vi "FibrePhotometry.vi"() -> ()   [LabVIEW 2016]
uses:
  <vilib>/DAQmx/read.llb/DAQmx Read (Analog 2D DBL NChan NSamp).vi
  <vilib>/DAQmx/write.llb/DAQmx Write (Analog 1D DBL NChan 1Samp).vi
  <vilib>/DAQmx/miscellaneous.llb/DAQmx Fill In Error Info.vi
  <vilib>/Utility/file.llb/Write Delimited Spreadsheet (DBL).vi
  <vilib>/DAQmx/create/channels.llb/DAQmx Create Channel (AO-Voltage-Basic).vi
panel:
  out "Start Time":u32
  in  "Recording":bool
  out "Recording Time":dbl
  out "Save Path":path
  out "Data":dbl[][](graph)
  out "Waveform":waveform(dbl)[](graph)
  in  "stop":bool
  out "Loop Time":u32
  in  "Comments":string
  in  "Dir":string="C:\\Test"
  in  "Raw samples per s":dbl=2000.0 min=2000.0 max=2000.0
  in  "405 LED Power":dbl=1.0 min=0.0 max=5.0
  in  "470 LED power":dbl=2.0 min=0.0 max=5.0
  in  "Frequency":dbl=10.0
  in  "Duty cycle (%)":dbl=40.0
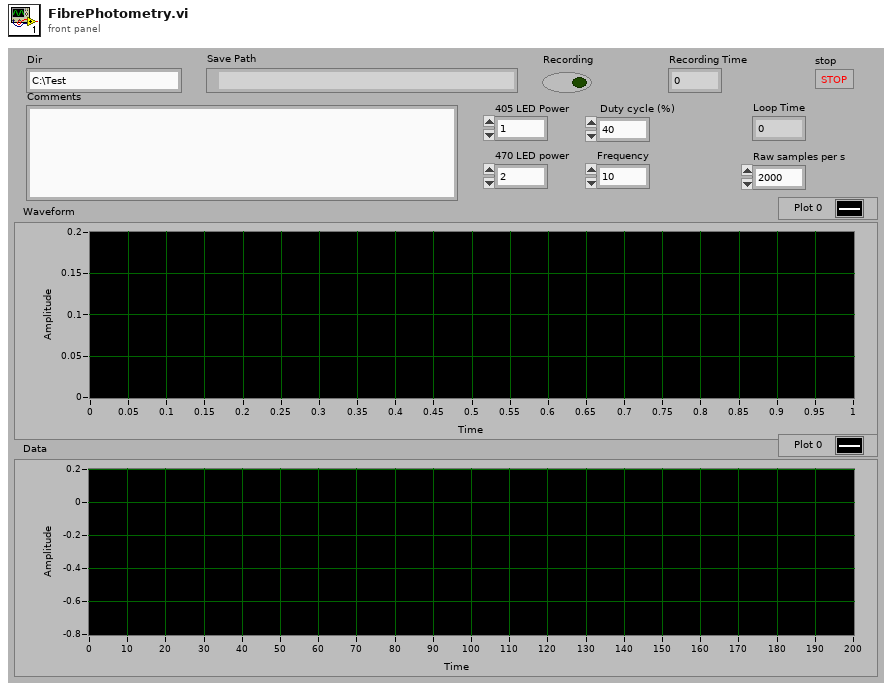
[diagram p1: front panel]
types:
  T1 = enum16{"big-endian, network order", "native, host order", "little-endian"}
  T2 = cluster{"Comments":string, "Dir":string, "Frequency":dbl, "470 LED power":dbl, "405 LED Power":dbl, "Raw samples per s":dbl, " Duty cycle (%)":dbl}
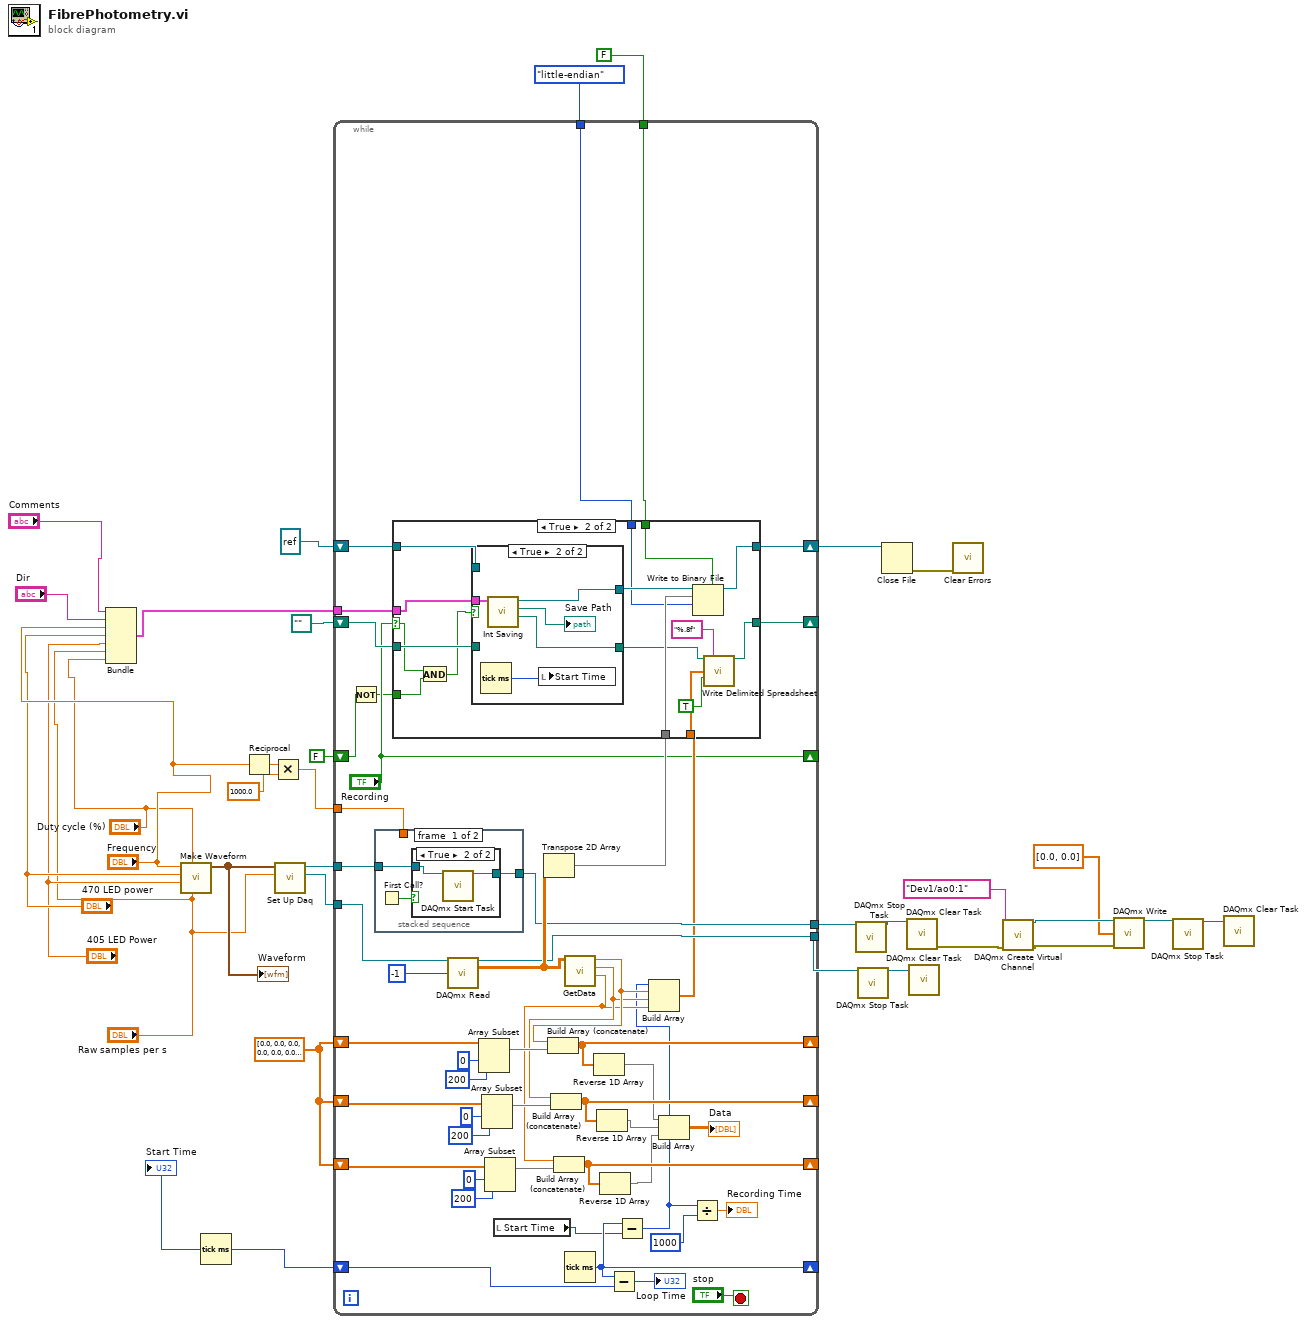
[diagram p0: block diagram]
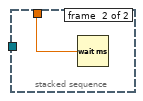
[diagram p5: hidden frame]
diagram:
  w23 = dbl[] [0.0, 0.0, 0.0, 0.0, 0.0, 0.0, 0.0, 0.0, 0.0, 0.0, 0.0, 0.0, 0.0, 0.0, 0.0, 0.0, 0.0, 0.0, 0.0, 0.0, 0.0, 0.0, 0.0, 0.0, 0.0, 0.0, 0.0, 0.0, 0.0, 0.0, 0.0, 0.0, 0.0, 0.0, 0.0, 0.0, 0.0, 0.0, 0.0, 0.0, 0.0, 0.0, 0.0, 0.0, 0.0, 0.0, 0.0, 0.0, 0.0, 0.0, 0.0, 0.0, 0.0, 0.0, 0.0, 0.0, 0.0, 0.0, 0.0, 0.0, 0.0, 0.0, 0.0, 0.0, 0.0, 0.0, 0.0, 0.0, 0.0, 0.0, 0.0, 0.0, 0.0, 0.0, 0.0, 0.0, 0.0, 0.0, 0.0, 0.0, 0.0, 0.0, 0.0, 0.0, 0.0, 0.0, 0.0, 0.0, 0.0, 0.0, 0.0, 0.0, 0.0, 0.0, 0.0, 0.0, 0.0, 0.0, 0.0, 0.0, 0.0, 0.0, 0.0, 0.0, 0.0, 0.0, 0.0, 0.0, 0.0, 0.0, 0.0, 0.0, 0.0, 0.0, 0.0, 0.0, 0.0, 0.0, 0.0, 0.0, 0.0, 0.0, 0.0, 0.0, 0.0, 0.0, 0.0, 0.0, 0.0, 0.0, 0.0, 0.0, 0.0, 0.0, 0.0, 0.0, 0.0, 0.0, 0.0, 0.0, 0.0, 0.0, 0.0, 0.0, 0.0, 0.0, 0.0, 0.0, 0.0, 0.0, 0.0, 0.0, 0.0, 0.0, 0.0, 0.0, 0.0, 0.0, 0.0, 0.0, 0.0, 0.0, 0.0, 0.0, 0.0, 0.0, 0.0, 0.0, 0.0, 0.0, 0.0, 0.0, 0.0, 0.0, 0.0, 0.0, 0.0, 0.0, 0.0, 0.0, 0.0, 0.0, 0.0, 0.0, 0.0, 0.0, 0.0, 0.0, 0.0, 0.0, 0.0, 0.0, 0.0, 0.0, 0.0, 0.0, 0.0, 0.0, 0.0, 0.0, 0.0]
  n1 = Bundle("Comments"="Comments", "Dir"="Dir", "Frequency"="Frequency", "470 LED power"="470 LED power", "405 LED Power"="405 LED Power", "Raw samples per s"="Raw samples per s", "Duty cycle (%)"="Duty cycle (%)") -> (w6:T2)  [unwired: 1 in]
  n2 = call "Make Waveform.vi"("Number of samples per s"="Raw samples per s", "Duty cycle (%)"="Duty cycle (%)", "405 LED Power"="405 LED Power", "470 LED power"="470 LED power", "Frequency"="Frequency") -> ("Array"=w24:waveform(dbl)[])  [unwired: 6 in]
  "Waveform" <- w24
  n3 = Tick Count (ms)() -> (millisecond timer value=w26:u32)
  "Start Time" <- w26
  n4 = Reciprocal(x="Frequency") -> (1/x=w32:dbl)
  n5 = Multiply(x=w32, y=1000.0) -> (x*y=w30:dbl)
  n6 = call "Set Up Daq.vi"("Number of samples per s"="Raw samples per s", "Array"=w24) -> ("task out 2"=w33:refnum<k21>, "Refnum out"=w34:refnum<k21>)  [unwired: 8 in]
  n7 = while {
    tunnel: w34 -> [w83]
    tunnel: w33 -> [w81]
    tunnel: w30 -> [w82]
    shift-right: [w46] -> w2
    shift-left: refnum<file> refnum ("refnum out") -> [w47]
    tunnel: [w78] -> w25
    tunnel: [w77] -> w28
    shift-right: [w73] -> _
    shift-left: w23 -> [w72]
    shift-right: [w65] -> _
    shift-left: w23 -> [w62]
    shift-right: [w64] -> _
    shift-left: w23 -> [w63]
    shift-right: [w57] -> _
    shift-left: w26 -> [w58]
    tunnel: FALSE ("prepend array or string size? (T)") -> [w44]
    tunnel: T1."little-endian" ("byte order (0:big-endian, network order)") -> [w43]
    tunnel: w6 -> [w41]
    shift-right: [w40] -> _
    shift-left: path "" ("new file path (Not A Path if cancelled)") -> [w39]
    shift-right: ["Recording"] -> _
    shift-left: FALSE ("Recording") -> [w36]
    stop <- "stop" stop-if-true
    n8 = Not(x=w36) -> (.not. x?=w35:bool)
    n9 = stacked-sequence {
      tunnel: w83 -> [w110 _]
      tunnel: [w109 _] -> w77
      tunnel: w82 -> [_ w115]
      frame #0 {
        n10 = First Call?() -> (First Call?: T/F=w111:bool)
        n11 = case shown="True" w111 {
          tunnel: w110 -> [w112 w114]
          tunnel: [w112 w113] -> w109
          frame False {
          }
          frame True {
            n12 = call <vilib>:"DAQmx Start Task.vi"("task/channels in"=w114) -> ("task out"=w113:refnum<k21>)  [unwired: 13 in, 1 out]
          }
        }
      }
      frame #1 {
        n13 = Wait (ms)(milliseconds to wait=w115) -> ()  [unwired: 1 out]
      }
    }
    n14 = call-poly <vilib>:"DAQmx Read.vi"("task/channels in"=w81, "number of samples per channel"=-1) -> ("task out"=w78:refnum<k21>, "data"=w79:dbl[][])  [unwired: 11 in, 1 out]
    n15 = Array Subset(array=w72, index=0, length=200) -> (w74:dbl[])
    n16 = Array Subset(array=w62, index=0, length=200) -> (w69:dbl[])
    n17 = Array Subset(array=w63, index=0, length=200) -> (w66:dbl[])
    n18 = local read "Start Time"() -> (w38:u32)
    n19 = Transpose 2D Array(2D array=w79) -> (transposed array=w45:dbl[][])
    n20 = call "GetData.vi"("data"=w79) -> ("mean 405"=w53:dbl, "mean 470"=w54:dbl, "F470/F405"=w55:dbl)  [unwired: 8 in]
    n21 = Build Array (concatenate)(w55, w74) -> (w73:dbl[])
    n22 = Build Array (concatenate)(w54, w69) -> (w65:dbl[])
    n23 = Build Array (concatenate)(w53, w66) -> (w64:dbl[])
    n24 = Tick Count (ms)() -> (millisecond timer value=w57:u32)
    n25 = Reverse 1D Array(array=w73) -> (reversed array=w60:dbl[])
    n26 = Reverse 1D Array(array=w65) -> (reversed array=w61:dbl[])
    n27 = Reverse 1D Array(array=w64) -> (reversed array=w59:dbl[])
    n28 = Subtract(x=w57, y=w58) -> (x-y=→"Loop Time":u32)
    n29 = Subtract(x=w57, y=w38) -> (x-y=w50:u32)
    n30 = Build Array(w50, w55, w54, w53) -> (w42:dbl[])
    n31 = case shown="True" "Recording" {
      selector: "Recording" -> [_ w87]
      tunnel: w47 -> [w85 w101]
      tunnel: [w85 w99] -> w46
      tunnel: w45 -> [_ w98]
      tunnel: w44 -> [_ w97]
      tunnel: w43 -> [_ w96]
      tunnel: w42 -> [_ w93]
      tunnel: w41 -> [_ w92]
      tunnel: [w84 w90] -> w40
      tunnel: w39 -> [w84 w89]
      tunnel: w35 -> [_ w88]
      frame False {
      }
      frame True {
        n32 = And(x=w87, y=w88) -> (x .and. y?=w86:bool)
        n33 = case shown="True" w86 {
          tunnel: w101 -> [w103 _]
          tunnel: [w103 w108] -> w100
          tunnel: w92 -> [_ w107]
          tunnel: [w102 w105] -> w91
          tunnel: w89 -> [w102 _]
          frame False {
          }
          frame True {
            n34 = Tick Count (ms)() -> (millisecond timer value=w104:u32)
            n35 = call "Int Saving.vi"("Cluster"=w107) -> ("Data.txt"=w105:path, "created path"=→"Save Path":path, "Byte Stream File out"=w108:refnum<file>)  [unwired: 8 in]
            n36 = local write "Start Time"(w104) -> ()
          }
        }
        n37 = Write to Binary File(file (use dialog)=w100, data=w98, 5:w97, 9:w96) -> (refnum out=w99:refnum<file>)  [unwired: 2 in, 2 out]
        n38 = call-poly <vilib>:"Write Delimited Spreadsheet.vi"("file path (dialog if empty)"=w91, "format (%.3f)"="%.8f", "1D data"=w93, "append to file? (new file:F)"=TRUE) -> ("new file path (Not A Path if cancelled)"=w90:path)  [unwired: 10 in, 1 out]
      }
    }
    n39 = Build Array(w60, w61, w59) -> (→"Data":dbl[][])
    n40 = Divide(x=w50, y=u32 1000) -> (x/y=→"Recording Time":dbl)
  }
  n41 = call <vilib>:"DAQmx Stop Task.vi"("task/channels in"=w28) -> ("task out"=w29:refnum<k21>)  [unwired: 13 in, 1 out]
  n42 = call <vilib>:"DAQmx Stop Task.vi"("task/channels in"=w25) -> ("task out"=w27:refnum<k21>)  [unwired: 13 in, 1 out]
  n43 = Close File(refnum=w2) -> (error out=w1:errorcluster)  [unwired: 1 in, 1 out]
  n44 = call <vilib>:"DAQmx Clear Task.vi"("task in"=w29) -> ("error out"=w22:errorcluster)  [unwired: 14 in]
  n45 = call <vilib>:"DAQmx Clear Task.vi"("task in"=w27) -> ()  [unwired: 14 in, 1 out]
  n46 = call <vilib>:"Clear Errors.vi"("error in (no error)"=w1) -> ()  [unwired: 5 in, 2 out]
  n47 = call-poly <vilib>:"DAQmx Create Virtual Channel.vi"("physical channels"=tag "Dev1/ao0:1", "error in"=w22) -> ("task out"=w19:refnum<k21>, "error out"=w20:errorcluster)  [unwired: 12 in]
  n48 = call-poly <vilib>:"DAQmx Write.vi"("task/channels in"=w19, "data"=dbl[] [0.0, 0.0], "error in"=w20) -> ("task out"=w16:refnum<k21>)  [unwired: 10 in, 2 out]
  n49 = call <vilib>:"DAQmx Stop Task.vi"("task/channels in"=w16) -> ("task out"=w17:refnum<k21>)  [unwired: 13 in, 1 out]
  n50 = call <vilib>:"DAQmx Clear Task.vi"("task in"=w17) -> ()  [unwired: 14 in, 1 out]
